vi "GPS_pcan.vi"(11 "GPS data":u8[][](array[numeric]) format="%.0x") -> (3 "GPS data 2":u8[](array[numeric]))   [LabVIEW 2024, in "PCANusb_DTU.lvlib"]
uses:
  PCANusb_DTU.lvlib
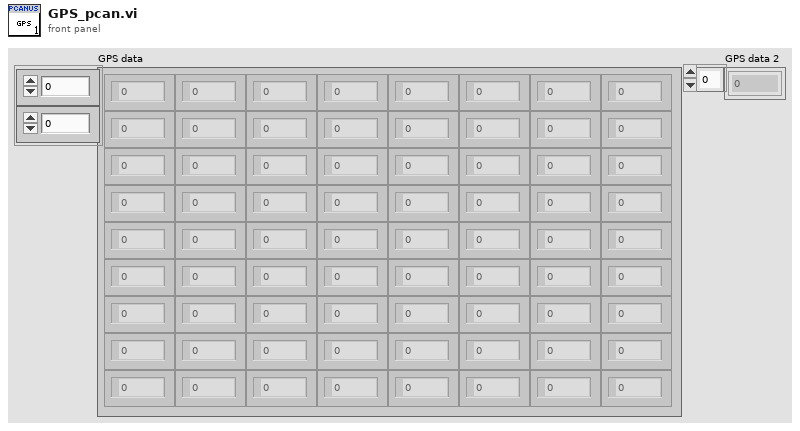
[diagram p1: front panel]
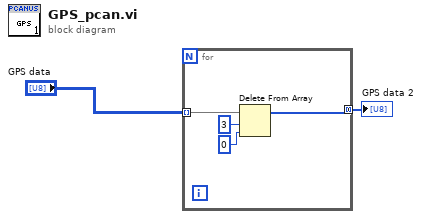
[diagram p0: block diagram]
diagram:
  n1 = for {
    tunnel: "GPS data" -> [w6] mode=indexing
    tunnel: [w3] -> w1 mode=concatenating
    n2 = Delete From Array(array=w6, length=3, index=0) -> (array with subset deleted=w3:u8[])  [unwired: 1 out]
  }
  "GPS data 2" <- w1
